vi "Time Control.vi"(10 "Action":u16(ring) items=["Start", "Stop", "No Action"], 11 "LabVIEW Web Service Request":refnum<class "Web Request.lvclass">) -> (0 "RemainingString":string, 1 "TimeRemaining":dbl, 2 "TimerRunning":bool)   [LabVIEW 2013]
uses:
  <vilib>/wsapi/Web Request.lvclass
  <vilib>/xml/Close Reference(Node).vi
  <vilib>/xml/NI_XML.lvlib
  <resource>/objmgr/DOMUserDefRef.rc
panel:
  out "MatchState":T1(ring)
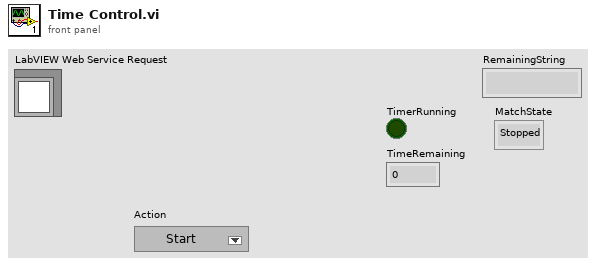
[diagram p1: front panel]
types:
  T1 = enum16{"Stopped", "Primary", "Secondary", "Pre-Primary"}
  T2 = enum16{"Get", "Increment", "Decrement", "Set Match", "Set Phase"}
  T3 = enum16{"Get Timer State", "Start Timer", "Stop Timer"}
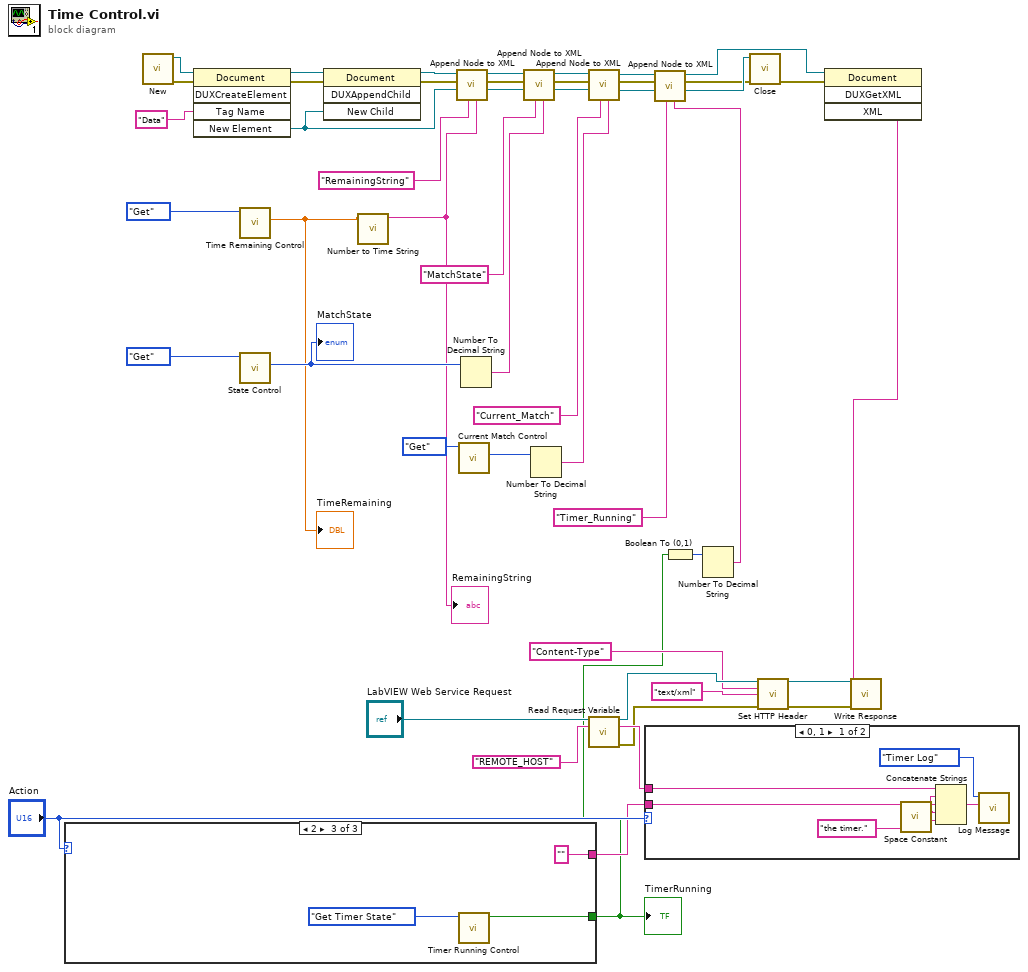
[diagram p0: block diagram]
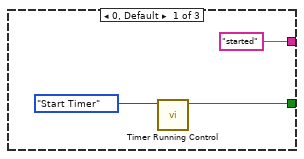
[diagram p3: hidden frame]
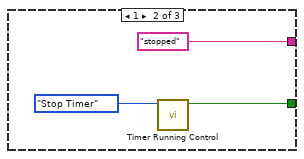
[diagram p4: hidden frame]
diagram:
  n1 = case shown="2" "Action" {
    tunnel: [w50 w53 w57] -> w5
    tunnel: ["started" "stopped" ""] -> w37
    frame 0, Default {
      n2 = call "Timer Running Control.vi"("Enum"=T3."Start Timer") -> ("Timer State"=w50:bool)  [unwired: 10 in]
    }
    frame 1 {
      n3 = call "Timer Running Control.vi"("Enum"=T3."Stop Timer") -> ("Timer State"=w53:bool)  [unwired: 10 in]
    }
    frame 2 {
      n4 = call "Timer Running Control.vi"("Enum"=T3."Get Timer State") -> ("Timer State"=w57:bool)  [unwired: 10 in]
    }
  }
  "TimerRunning" <- w5
  n5 = call <vilib>:"New.vi"() -> ("error out"=w48:errorcluster, "DOM document out"=w49:refnum<k20>)  [unwired: 8 in]
  n6 = invoke class="Document" method="DUXCreateElement"(reference=w49, error in=w48, "Tag Name"="Data") -> (reference out=w46:refnum<k20>, error out=w45:errorcluster, "New Element"=w33:refnum<k20>)  [unwired: 2 in, 2 out]
  n7 = call "Time Remaining Control.vi"("Mode"=enum16{"Get", "Set"}."Get") -> ("Time Remaining"=w2:dbl)  [unwired: 10 in]
  "TimeRemaining" <- w2
  n8 = call "State Control.vi"("Action"=enum16{"Get", "Set"}."Get") -> ("State Out"=w21:T1)  [unwired: 10 in]
  "MatchState" <- w21
  n9 = invoke class="Document" method="DUXAppendChild"(reference=w46, error in=w45, "New Child"=w33) -> (reference out=w44:refnum<k20>, error out=w43:errorcluster)  [unwired: 1 in, 2 out]
  n10 = call "Number to Time String.vi"("Numeric"=w2) -> ("String"=w1:string)  [unwired: 10 in]
  "RemainingString" <- w1
  n11 = call "Append Node to XML.vi"("Data"=w1, "Tag Name"="RemainingString", "SuperElement In"=w33, "error in"=w43, "DOM document in"=w44) -> ("SuperElement Out"=w31:refnum<k20>, "error out"=w41:errorcluster, "DOM document out"=w42:refnum<k20>)  [unwired: 4 in]
  n12 = call "Current Match Control.vi"("Mode"=T2."Get") -> ("Current Match"=w15:u16)  [unwired: 9 in, 1 out]
  n13 = Number To Decimal String(number=w21) -> (decimal integer string=w29:string)  [unwired: 1 in]
  n14 = call "Append Node to XML.vi"("Data"=w29, "Tag Name"="MatchState", "SuperElement In"=w31, "error in"=w41, "DOM document in"=w42) -> ("SuperElement Out"=w18:refnum<k20>, "error out"=w17:errorcluster, "DOM document out"=w19:refnum<k20>)  [unwired: 4 in]
  n15 = Number To Decimal String(number=w15) -> (decimal integer string=w14:string)  [unwired: 1 in]
  n16 = call "Append Node to XML.vi"("Data"=w14, "Tag Name"="Current_Match", "SuperElement In"=w18, "error in"=w17, "DOM document in"=w19) -> ("SuperElement Out"=w10:refnum<k20>, "error out"=w11:errorcluster, "DOM document out"=w12:refnum<k20>)  [unwired: 4 in]
  n17 = call <vilib>:"Read Request Variable.vi"("LabVIEW Web Service Request"="LabVIEW Web Service Request", "variable name"="REMOTE_HOST") -> ("LabVIEW Web Service Request out"=w28:refnum<class "Web Request.lvclass">, "value"=w34:string, "error out"=w25:errorcluster)  [unwired: 11 in]
  n18 = case shown="0, 1" "Action" {
    tunnel: w37 -> [w63 _]
    tunnel: w34 -> [w61 _]
    frame 0, 1 {
      n19 = call <vilib>:"Space Constant.vi"() -> ("String"=w60:string)
      n20 = Concatenate Strings(w61, w60, w63, w60, "the timer." ("string")) -> (w64:string)
      n21 = call "Log Message.vi"("Message"=w64, "Log"=enum16{"Error Log", "Timer Log", "Scoring Log"}."Timer Log") -> ()  [unwired: 10 in]
    }
    frame Default {
    }
  }
  n22 = Boolean To (0,1)(Boolean=w5) -> (0, 1=w4:i16)
  n23 = Number To Decimal String(number=w4) -> (decimal integer string=w3:string)  [unwired: 1 in]
  n24 = call "Append Node to XML.vi"("Data"=w3, "Tag Name"="Timer_Running", "SuperElement In"=w10, "error in"=w11, "DOM document in"=w12) -> ("SuperElement Out"=w9:refnum<k20>, "error out"=w8:errorcluster, "DOM document out"=w7:refnum<k20>)  [unwired: 4 in]
  n25 = call-poly <vilib>:"Close.vi"("error in (no error)"=w8, "node"=w9) -> ("error out"=w40:errorcluster)  [unwired: 7 in]
  n26 = call <vilib>:"Set HTTP Header.vi"("LabVIEW Web Service Request"=w28, "header"="Content-Type", "header value"="text/xml", "error in (no error)"=w25) -> ("LabVIEW Web Service Request out"=w27:refnum<class "Web Request.lvclass">, "error out"=w26:errorcluster)  [unwired: 10 in]
  n27 = invoke class="Document" method="DUXGetXML"(reference=w7, error in=w40) -> ("XML"=w39:string)  [unwired: 2 in, 3 out]
  n28 = call <vilib>:"Write Response.vi"("LabVIEW Web Service Request"=w27, "response string"=w39, "error in (no error)"=w26) -> ()  [unwired: 11 in, 2 out]
